vi "RSQ_COD_exercise_subvi.vi"(10 "Data Yi's":dbl[](array[numeric]), 11 "Model fi's":dbl[](array[numeric])) -> (3 "COD-RSQ":dbl)   [LabVIEW 2019]
uses:
  <vilib>/Analysis/baseanly.llb/Mean (DBL).vi
  <vilib>/Analysis/NI_AALBase.lvlib
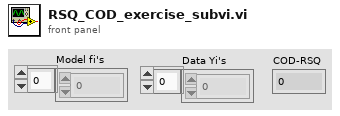
[diagram p1: front panel]
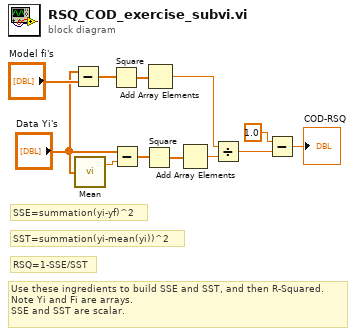
[diagram p0: block diagram]
diagram:
  # "RSQ=1-SSE/SST"
  # "SST=summation(yi-mean(yi))^2"
  # "SSE=summation(yi-yf)^2"
  # "Use these ingredients to build SSE and SST, and then R-Squared.\nNote Yi and Fi are arrays.\nSSE and SST are scalar."
  n1 = Subtract(x="Data Yi's", y="Model fi's") -> (x-y=w11:dbl[])
  n2 = call-poly <vilib>:"Mean.vi"("X"="Data Yi's") -> ("mean"=w8:dbl)  [unwired: 1 out]
  n3 = Square(x=w11) -> (x^2=w10:dbl[])
  n4 = Subtract(x="Data Yi's", y=w8) -> (x-y=w6:dbl[])
  n5 = Square(x=w6) -> (x^2=w7:dbl[])
  n6 = Add Array Elements(numeric array=w10) -> (sum=w5:dbl)
  n7 = Add Array Elements(numeric array=w7) -> (sum=w4:dbl)
  n8 = Divide(x=w5, y=w4) -> (x/y=w3:dbl)
  n9 = Subtract(x=1.0, y=w3) -> (x-y=→"COD-RSQ":dbl)
